vi "Status.vi"(10 "error in (no error)":errorcluster, 11 "System Config Status API in":refnum<class "System Config Status API.lvclass">) -> (2 "error out":errorcluster, 3 "Config Status":T1[](array[typedef]))   [LabVIEW 2020, in "Volatus.lvlib" / "System Config Status API.lvclass"]
uses:
  System Config Status API.lvclass
  System Config Status API.lvclass/System Config Status API.ctl
  Config Alert Module/Node Config Info.ctl
  Volatus.lvlib
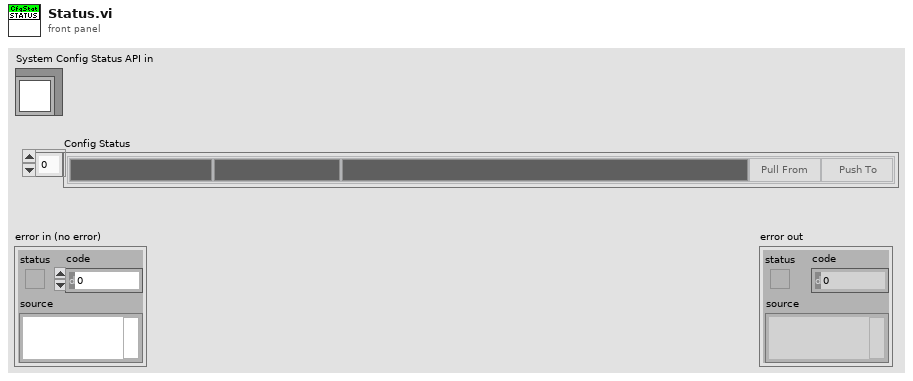
[diagram p1: front panel]
types:
  T1 = typedef "Volatus.lvlib/Node Config Info.ctl" = cluster{"Node":string, "Config Version":string, "Config Hash":string, "Pull":bool, "Push":bool, "Version Color":u32, "Hash Color":u32, "Node Color":u32}
  T2 = typedef "Volatus.lvlib/Config Monitor Module.lvclass/Node Config Info.ctl" = cluster{"Node":string, "Config Version":string, "Config Hash":string, "Pull":bool, "Push":bool, "Version Color":u32, "Hash Color":u32, "Node Color":u32}
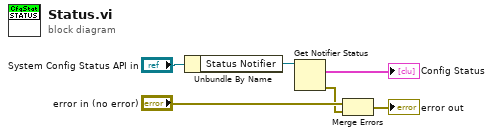
[diagram p0: block diagram]
diagram:
  n1 = Unbundle By Name("System Config Status API in") -> ("Status Notifier"=w4:refnum<notifier>)
  n2 = Get Notifier Status(notifier=w4) -> (current notification=→"Config Status":T2[], error out=w1:errorcluster)  [unwired: 1 in, 3 out]
  n3 = Merge Errors("error in (no error)", w1) -> (→"error out":errorcluster)
